vi "Unpack for gRPC.vi"(8 "error in (no error)":errorcluster, 9 "Configuration / Resuls (Config)":enum16{"Configuration", "Results"}(ring), 10 "Any":T1, 11 "Measurement Customizations in":refnum<class "MeasurementPlugin.lvclass">) -> (0 "error out":errorcluster, 2 "Data Value":variant, 3 "Measurement Customizations out":refnum<class "MeasurementPlugin.lvclass">)   [LabVIEW 2021, in "Channel To Channel Isolation_ADC.lvlib" / "MeasurementPlugin.lvclass"]
uses:
  MeasurementPlugin.lvclass
  <vilib>/gRPC/LabVIEW gRPC Library/Shared/Any.ctl
  C:/Program Files/National Instruments/LabVIEW 2021/vi.lib/MeasurementLink/MeasurementLink Measurement Server/Measurement Plugin Service/Measurement Plugin Service.lvclass
  Measurement Configuration.ctl
  Measurement Results.ctl
  a521b266-ce99-437c-923d-067dcf1e07fd.vi
  3ecd018e-d556-4cbc-bc60-c4ba57204520.vi
  <vilib>/gRPC/LabVIEW gRPC Library/Server API/Translate Protobuf Error.vi
  <vilib>/AdvancedString/1D String Array to Delimited String.vi
  <vilib>/gRPC/LabVIEW gRPC Library/Server API/Server/Get Server DLL Path.vi
  Channel To Channel Isolation_ADC.lvlib
  <vilib>/MeasurementLink/MeasurementLink Measurement Server/Measurement Plugin Service/Measurement Plugin Service.lvclass
  <vilib>/gRPC/LabVIEW gRPC Library/grpc-lvsupport-release.lvlib
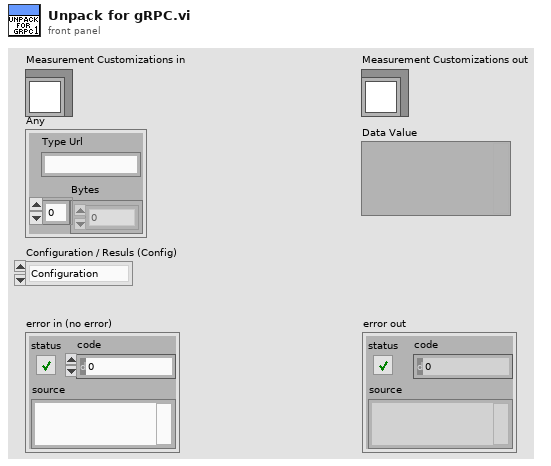
[diagram p1: front panel]
types:
  T1 = typedef "grpc-lvsupport-release.lvlib/Any.ctl" = cluster{"Type Url":string, "Bytes":u8[]}
  T2 = typedef "grpc-lvsupport-release.lvlib/grpcId.ctl" = u64
  T3 = typedef "Channel To Channel Isolation_ADC.lvlib/Measurement Configuration.ctl" = cluster{"Victim channel":i32, "Full scale range":dbl, "Interferer channels":i32[], "Victim channel resource name":string, "Victim frequency":dbl, "Victim amplitude":dbl, "Interferer channel resource name":string, "Interferer channel channel":i32, "Interferer start frequency":dbl, "Interferer stop frequency":dbl, "Interferer number of steps":i32, "Interferer sweep type":u32, "Interferer amplitude":dbl, "Digital capture resource name":string, "Digital capture sample rate":dbl, "Digital capture samples":u32}
  T4 = typedef "Channel To Channel Isolation_ADC.lvlib/Measurement Results.ctl" = cluster{"Victim channel name":string, "Crosstalk":dbl, "Frequency":dbl, "Frequency waveform":dbl[], "Crosstalk waveform":dbl[], "f0":dbl, "df":dbl, "Spectrum":dbl[], "Spectrum plot size":i32, "t0":dbl, "dt":dbl, "Time domain":dbl[], "Time domain plot size":i32}
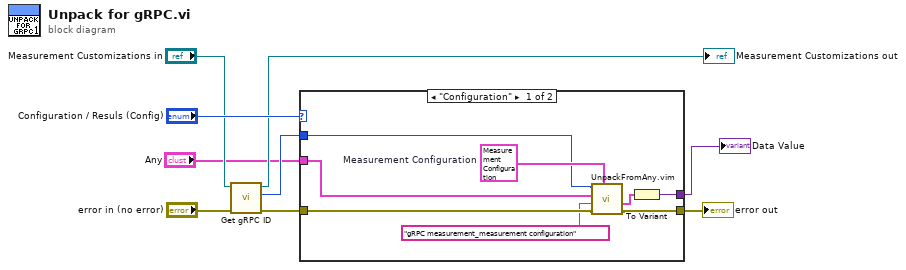
[diagram p0: block diagram]
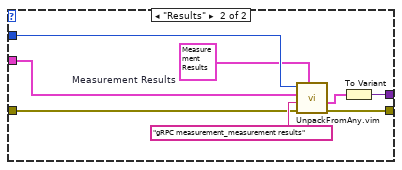
[diagram p2: hidden frame]
diagram:
  n1 = call <vilib>:"Get gRPC ID.vi"("error in"="error in (no error)", "measurement plugin service in"="Measurement Customizations in") -> ("error out"=w6:errorcluster, "gRPC ID"=w3:T2, "measurement plugin service out"=→"Measurement Customizations out":refnum<class "MeasurementPlugin.lvclass">)  [unwired: 7 in]
  n2 = case shown="\"Configuration\"" "Configuration / Resuls (Config)" {
    tunnel: w6 -> [w15 w19]
    tunnel: "Any" -> [w10 w18]
    tunnel: w3 -> [w12 w22]
    tunnel: [w16 w23] -> w9
    tunnel: [w17 w25] -> w1
    frame "Configuration" {
      w13 = T3 {"Victim channel"=0, "Full scale range"=10.0, "Interferer channels"=[2], "Victim channel resource name"="", "Victim frequency"=-1.0, "Victim amplitude"=1000.0, "Interferer channel resource name"="", "Interferer channel channel"=0, "Interferer start frequency"=100000.0, "Interferer stop frequency"=160000.0, "Interferer number of steps"=10, "Interferer sweep type"=0, "Interferer amplitude"=-1.0, "Digital capture resource name"="", "Digital capture sample rate"=800000.0, "Digital capture samples"=800000}  # Measurement Configuration
      n3 = call "UnpackFromAny.vim"("Data Type"=w13, "error in"=w15, "Message Type"="gRPC measurement_measurement configuration", "Any"=w10, "gRPCid in"=w12) -> ("error out"=w16:errorcluster, "Unpacked Value"=w14:T3)  [unwired: 4 in, 1 out]
      n4 = To Variant(anything=w14) -> (Variant=w17:variant)
    }
    frame "Results" {
      w21 = T4 {"Victim channel name"="", "Crosstalk"=0.0, "Frequency"=0.0, "Frequency waveform"=[], "Crosstalk waveform"=[], "f0"=0.0, "df"=0.0, "Spectrum"=[], "Spectrum plot size"=0, "t0"=0.0, "dt"=0.0, "Time domain"=[], "Time domain plot size"=0}  # Measurement Results
      n5 = call "UnpackFromAny.vim"("Data Type"=w21, "error in"=w19, "Message Type"="gRPC measurement_measurement results", "Any"=w18, "gRPCid in"=w22) -> ("error out"=w23:errorcluster, "Unpacked Value"=w24:T4)  [unwired: 4 in, 1 out]
      n6 = To Variant(anything=w24) -> (Variant=w25:variant)
    }
  }
  "error out" <- w9
  "Data Value" <- w1
